vi "FPGA_MAin.vi"(0 "Aromi Pump Enable":bool, 1 "Aromi Pump":bool, 2 "Aromi LED":bool, 3 "Kiuas LED":bool, 5 "Löyly Valve":bool, 7 "Löyly Valve Enable":bool, 9 "Löyly LED":bool, 11 "Pump Enable":bool, 12 "Pump Direction":bool, 14 "Pump Cycle":u32 caption="Count(uSec)") -> (4 "Kiuas Switch":bool, 6 "Aromi Switch":bool, 8 "Löyly Switch":bool)   [LabVIEW 2019]
uses:
  <vilib>/eio/EIONode/EIONode.xnode
  <vilib>/rvi/eio/common/nirviEmuTemplateMethod_errors.vi
  <vilib>/eio/EIOMethodNode/EIOMethodNode.xnode
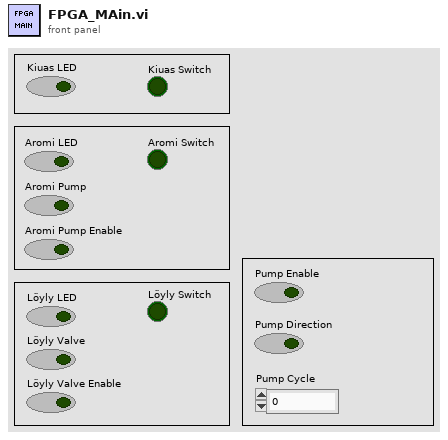
[diagram p1: front panel]
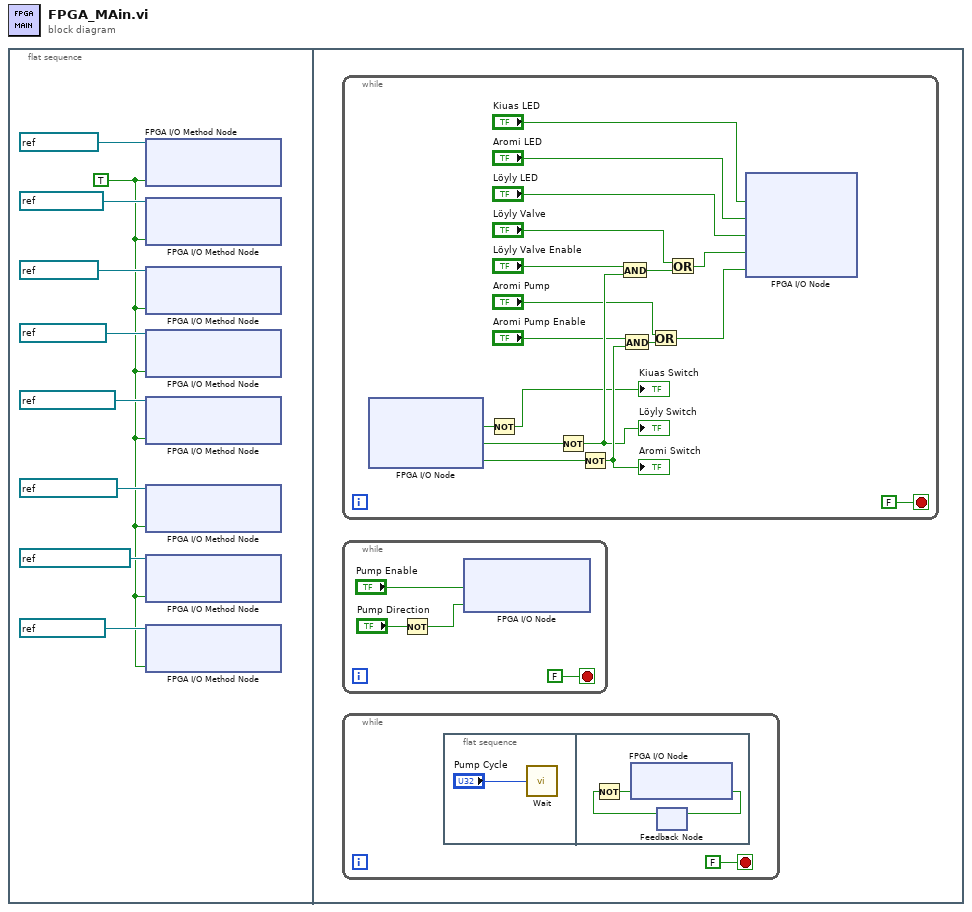
[diagram p0: block diagram]
diagram:
  n1 = flat-sequence {
    frame #0 {
      w1 = TRUE ("Enable")
      n2 = xnode "FPGA I/O Method Node"("FPGA I/O In"=refnum<k21> "Kiuas LED" ("FPGA I/O"), "Enable"=w1) -> ()  [unwired: 1 out]
      n3 = xnode "FPGA I/O Method Node"("FPGA I/O In"=refnum<k21> "Aromi LED" ("FPGA I/O"), "Enable"=w1) -> ()  [unwired: 1 out]
      n4 = xnode "FPGA I/O Method Node"("FPGA I/O In"=refnum<k21> "Löyly LED" ("FPGA I/O"), "Enable"=w1) -> ()  [unwired: 1 out]
      n5 = xnode "FPGA I/O Method Node"("FPGA I/O In"=refnum<k21> "Löyly Valve" ("FPGA I/O"), "Enable"=w1) -> ()  [unwired: 1 out]
      n6 = xnode "FPGA I/O Method Node"("FPGA I/O In"=refnum<k21> "Aromi Pump" ("FPGA I/O"), "Enable"=w1) -> ()  [unwired: 1 out]
      n7 = xnode "FPGA I/O Method Node"("FPGA I/O In"=refnum<k21> "Pump Enable" ("FPGA I/O"), "Enable"=w1) -> ()  [unwired: 1 out]
      n8 = xnode "FPGA I/O Method Node"("FPGA I/O In"=refnum<k21> "Pump Direction" ("FPGA I/O"), "Enable"=w1) -> ()  [unwired: 1 out]
      n9 = xnode "FPGA I/O Method Node"("FPGA I/O In"=refnum<k21> "Pump Step" ("FPGA I/O"), "Enable"=w1) -> ()  [unwired: 1 out]
    }
    frame #1 {
      n10 = while {
        stop <- FALSE stop-if-true
        n11 = xnode "FPGA I/O Node"() -> ("Kiuas Switch"=w33:bool, "Löyly Switch"=w23:bool, "Aromi Switch"=w32:bool)  [unwired: 3 in, 3 out]
        n12 = Not(x=w33) -> (.not. x?=→"Kiuas Switch":bool)
        n13 = Not(x=w23) -> (.not. x?=w27:bool)
        "Löyly Switch" <- w27
        n14 = Not(x=w32) -> (.not. x?=w30:bool)
        "Aromi Switch" <- w30
        n15 = And(x="Löyly Valve Enable", y=w27) -> (x .and. y?=w28:bool)
        n16 = And(x="Aromi Pump Enable", y=w30) -> (x .and. y?=w29:bool)
        n17 = Or(x="Aromi Pump", y=w29) -> (x .or. y?=w25:bool)
        n18 = Or(x="Löyly Valve", y=w28) -> (x .or. y?=w20:bool)
        n19 = xnode "FPGA I/O Node"("Kiuas LED"="Kiuas LED", "Aromi LED"="Aromi LED", "Löyly LED"="Löyly LED", "Löyly Valve"=w20, "Aromi Pump"=w25) -> ()  [unwired: 5 in, 5 out]
      }
      n20 = while {
        stop <- FALSE stop-if-true
        n21 = Not(x="Pump Direction") -> (.not. x?=w14:bool)
        n22 = xnode "FPGA I/O Node"("Pump Enable"="Pump Enable", "Pump Direction"=w14) -> ()  [unwired: 2 in, 2 out]
      }
      n23 = while {
        stop <- FALSE stop-if-true
        n24 = flat-sequence {
          frame #0 {
            n25 = call "Wait"("Count(Ticks)"="Pump Cycle") -> ()  [unwired: 1 out]
          }
          frame #1 {
            n26 = feedback #1() -> (w13:bool)  [unwired: 1 in]
            n27 = Not(x=w13) -> (.not. x?=w12:bool)
            n28 = xnode "FPGA I/O Node"("Pump Step"=w12) -> ()  [unwired: 1 in, 1 out]
            n29 = feedback-in #1(w12) -> ()
          }
        }
      }
    }
  }
